vi "read_params.vi"(8 "error in (no error)":errorcluster, 11 "IncrementalPCA in":refnum<class "IncrementalPCA.lvclass">) -> (0 "error out":errorcluster, 2 "params":T1={"n_components"={"n_components_type"="None", "n_components_int"=0.0}, "whiten"=FALSE, "copy"=TRUE, "batch_size"={"batch_size_type"="None", "batch_size_int"=0.0}}, 3 "IncrementalPCA out":refnum<class "IncrementalPCA.lvclass">)   [LabVIEW 2020, in "IncrementalPCA.lvclass"]
uses:
  IncrementalPCA.lvclass
  Controls/incremental_pca_params.ctl
  IncrementalPCA.lvclass/IncrementalPCA.ctl
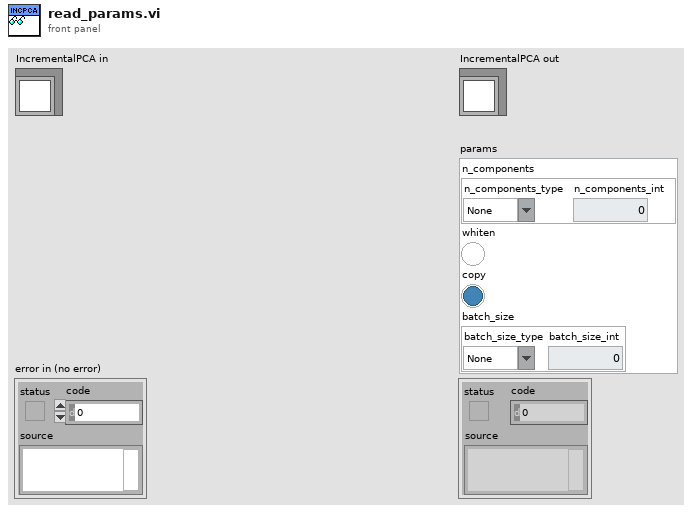
[diagram p1: front panel]
types:
  T1 = typedef "incremental_pca_params.ctl" = cluster{"n_components":cluster{"n_components_type":string, "n_components_int":dbl}, "whiten":bool, "copy":bool, "batch_size":cluster{"batch_size_type":string, "batch_size_int":dbl}}
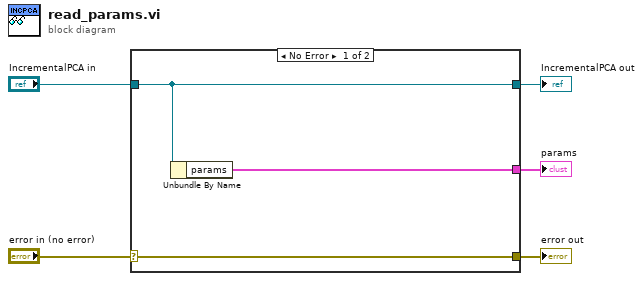
[diagram p0: block diagram]
diagram:
  n1 = case shown="No Error" "error in (no error)" {
    selector: "error in (no error)" -> [w8 w9]
    tunnel: [w8 w9] -> w4
    tunnel: [w7 w10] -> w2
    tunnel: "IncrementalPCA in" -> [w7 w10]
    tunnel: [w6 _] -> w1
    frame No Error {
      n2 = Unbundle By Name(w7) -> ("params"=w6:T1)
    }
    frame Error {
    }
  }
  "error out" <- w4
  "IncrementalPCA out" <- w2
  "params" <- w1
